vi "specu1a 1.0.0 Get TS from Variant array.vi"(1 "Array":cluster{variant}[](array[cluster]), 2 "Variant":variant) -> (0 "Numeric":i32)   [LabVIEW 2010]
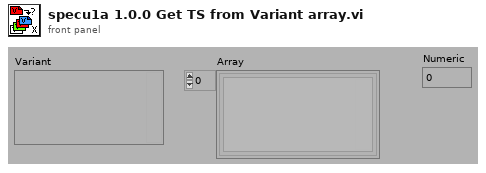
[diagram p1: front panel]
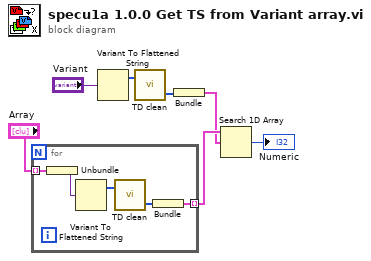
[diagram p0: block diagram]
diagram:
  n1 = for {
    tunnel: "Array" -> [w12] mode=indexing
    tunnel: [w8] -> w2 mode=indexing
    n2 = Unbundle(w12) -> (w11:variant)
    n3 = Variant To Flattened String(Variant=w11) -> (1:w10:i16[])  [unwired: 1 out]
    n4 = call "TD clean.vi"("type string in"=w10) -> ("Cleaned Type String out"=w9:i16[])  [unwired: 1 in, 1 out]
    n5 = Bundle("Cleaned Type String out"=w9) -> (w8:cluster{"Cleaned Type String out":i16[]})  [unwired: 1 in]
  }
  n6 = Variant To Flattened String(Variant="Variant") -> (1:w7:i16[])  [unwired: 1 out]
  n7 = call "TD clean.vi"("type string in"=w7) -> ("Cleaned Type String out"=w5:i16[])  [unwired: 1 in, 1 out]
  n8 = Bundle("Cleaned Type String out"=w5) -> (w1:cluster{"Cleaned Type String out":i16[]})  [unwired: 1 in]
  n9 = Search 1D Array(1D array=w2, element=w1) -> (index of element=→"Numeric":i32)  [unwired: 1 in]
